vi "ClearPathModeLists.vi"(0 "ClearActions":i32, 5 "error in":T1) -> (19 "error out":T1)   [LabVIEW 2016]
doc: "Clears the list of points saved in the path mode. If the variable \"ClearActions\" is set to 1, the action list will be cleared, too."
uses:
  Controls/Error_Out.ctl
  Files_ASC500/DLL/ASC500_RemoteControlV27.dll
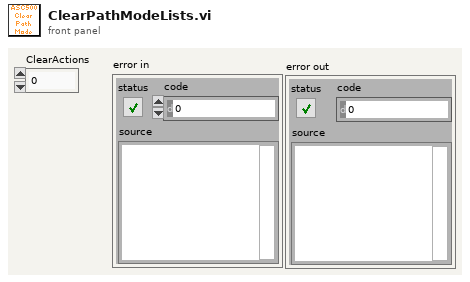
[diagram p1: front panel]
types:
  T1 = typedef "Error_Out.ctl" = errorcluster
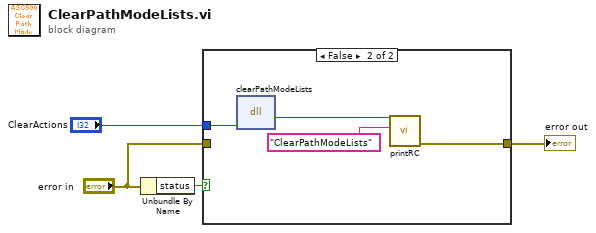
[diagram p0: block diagram]
diagram:
  n1 = Unbundle By Name("error in") -> ("status"=w4:bool)
  n2 = case shown="False" w4 {
    tunnel: [w5 w7] -> w2
    tunnel: "error in" -> [w5 _]
    tunnel: "ClearActions" -> [_ w6]
    frame True {
    }
    frame False {
      n3 = dll-call lib="G:/SCMOperations/Share/ELE/Produkt Information/ASC500/04 Remote Control/02 development versions/2018Nov06/Files_ASC500/DLL/ASC500_RemoteControlV27.dll" fn="clearPathModeLists"("ClearActions"=w6) -> ("return type"=w9:i32)  [unwired: 4 in, 2 out]
      n4 = call "printRC.vi"("additional information"="ClearPathModeLists", "RC"=w9) -> ("error out"=w7:T1)  [unwired: 9 in]
    }
  }
  "error out" <- w2
